vi "Driver.vi"(9 "Device Inputs FIFO":refnum<k33>, 10 "Device Outputs FIFO":refnum<k33>, 11 "Device Reference":T1 format="%.0x") -> ()   [LabVIEW 2023, in "NI 272x Resistive Simulation Custom Device Engine.lvlib"]
uses:
  NI 272x Resistive Simulation Custom Device Engine.lvlib
  <vilib>/NI VeriStand/Custom Device Tools/Custom Device Utility Library/Custom Device Utility Library.lvlib
  <vilib>/Platform/TimedLoop/XDataNode/XDataNode.xnode
  <vilib>/Platform/TimedLoop/XDataNode/nitl_modes.ctl
  <vilib>/Platform/TimedLoop/XDataNode/XDNodeRunTimeDep.lvlib
  <vilib>/Platform/TimedLoop/XDataNode/wakeup.ctl
  <vilib>/Platform/TimedLoop/XDataNode/timing_clust.ctl
  Controls/Connection control.ctl
  <vilib>/NI VeriStand/Custom Device API/Custom Device Item Ref.ctl
  <vilib>/NI VeriStand/Custom Device API/Custom Device API.lvlib
panel:
  in  "Initialization Status Notifier":refnum<notifier>
  in  "Status Notifier":refnum<notifier>
  # "Custom Device Template\nv1.0"
  # "Use this template as a starting point for creating a custom device code module. The input controls shown here are specially named controls that the system will use to provide the device loop with data. The controls are not required for the device loop to run. For instance, if the device doesn't produce any output data, then you don't need the Device Outputs FIFO control. If you do use these controls, however, they need to have these exact names to be functional."
  # "The optional status notifier element is used to notify the RT engine of the last state of the custom device, and to indicate the device has completed execution. If this control is not used, a default No Error value is returned to the system when the device finishes execution.\n\nNote: This error state is not checked until the system shuts down. Use an output status channel to send more immediate status values to the system."
  # "This optional input can be used to send the VeriStand Engine the final status of the custom device initalization process. If this control exists on the custom device front panel, the VeriStand Engine will wait for a status update before starting up. If the custom device reports an error, that will abort the execution of the current configuration in the VeriStand Engine.\n\nThis control can be deleted if the custom device does not need to send the initialization status update."
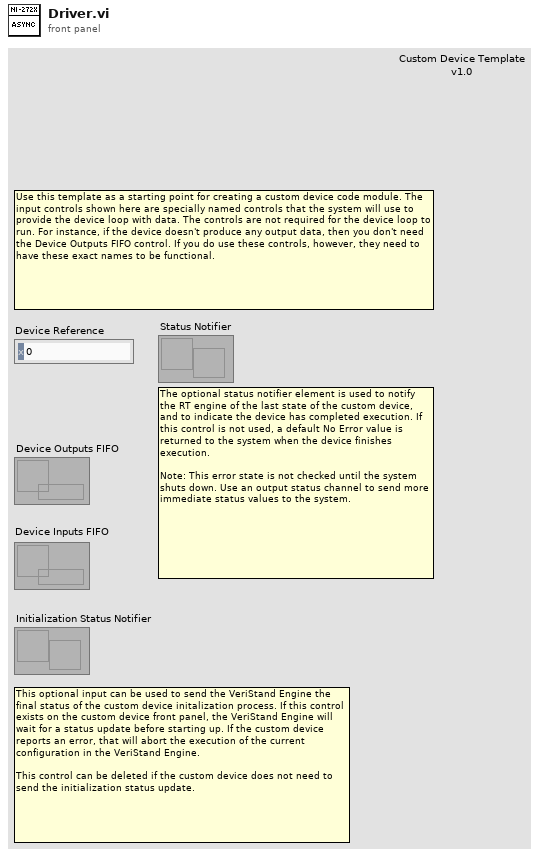
[diagram p1: front panel]
types:
  T1 = typedef "Custom Device API.lvlib/Custom Device Item Ref.ctl" = u64
  T2 = typedef "NI 272x Resistive Simulation Custom Device Engine.lvlib/Connection control.ctl" = enum16{"Connect (First Iter Only)", "Disconnect"}
  T3 = typedef "NI 272x Resistive Simulation Custom Device Engine.lvlib/Engine Run Time Data.ctl" = cluster{"Compiled Engine Data":T4, "CD In Buf":dbl[], "CD Out Buf":dbl[], "Device Outputs FIFO":refnum<k33>, "Device Inputs FIFO":refnum<k33>, "Instr":T9, "FirstIter":bool}
  T4 = typedef "NI 272x Resistive Simulation Custom Device Shared.lvlib/Compiled Engine Data.ctl" = cluster{"HW Chns":T5[], "Con Chns":T8[], "Err Idx":i32, "Late Idx":i32, "Dur Idx":i32, "DevName":string, "CD In Size":i32, "CD Out Size":i32, "TL dt":i64}
  T5 = typedef "NI 272x Resistive Simulation Custom Device Shared.lvlib/Compiled HW Channel.ctl" = cluster{"Mode":T6, "RTD":T7, "Desired Idx":i32, "Actual Idx":i32, "Last Des Val":dbl, "HW CH":string}
  T6 = typedef "NI 272x Resistive Simulation Custom Device Shared.lvlib/Channel Mode.ctl" = enum16{"Resistance", "RTD Temperature"}
  T7 = typedef "ni272x Callendar-Van Dusen RTD Parameters.ctl" = cluster{"A":dbl, "B":dbl, "C":dbl, "R0":dbl}
  T8 = typedef "NI 272x Resistive Simulation Custom Device Shared.lvlib/Compiled Connect Channel.ctl" = cluster{"Chn Idx":i32, "HW CH":string, "Is Con":bool, "HW CH+1":string}
  T9 = typedef "ni272x Reference.ctl" = refnum<k20>
  T10 = typedef "XDNodeRunTimeDep.lvlib/timing_clust.ctl" = cluster{"Expected End [f-1]":u64, "Actual End [f-1]":u64, "Finished Late? [f-1]":bool, "Expected End [i-1]":u64, "Actual End [i-1]":u64, "Finished Late? [i-1]":bool, "Expected Start [i]":u64, "Actual Start [i]":u64, "Expected Start [f]":u64, "Actual Start [f]":u64, "Source Name":string, "Structure Name":string, "Period":i64, "Deadline":i64, "Offset":i64, "Start":i64, "Priority":i32, "Timeout":i32, "Mode":T11, "Wakeup Reason":T12, "Error":errorcluster, "Source Type":string, "Secondary Source Type":string, "Global End Time":u64, "Global Start Time":u64, "Frame Duration":u64, "Iteration Duration":u64, "Assigned CPU":i32, "I/O Scan Engine Mode":u32}
  T11 = typedef "XDNodeRunTimeDep.lvlib/nitl_modes.ctl" = enum32{"No Change", "Process missed periods, maintain original phase", "Discard missed periods, maintain original phase", "Process missed periods, ignore original phase", "Discard missed periods, ignore original phase"}
  T12 = typedef "XDNodeRunTimeDep.lvlib/wakeup.ctl" = enum32{"Normal", "Aborted", "Asynchronous wakeup", "Timing source error", "Timed loop error", "Timeout"}
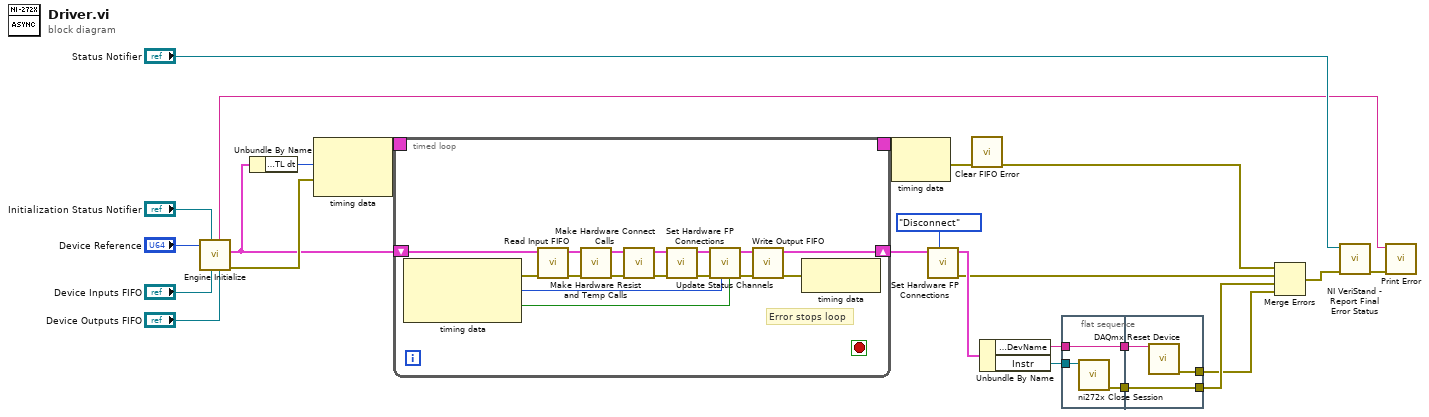
[diagram p0: block diagram]
diagram:
  n1 = call "Engine Initialize.vi"("Device Outputs FIFO"="Device Outputs FIFO", "Device Inputs FIFO"="Device Inputs FIFO", "Initialization Status Notifier"="Initialization Status Notifier", "Device Reference"="Device Reference") -> ("error out"=w19:errorcluster, "Engine Run Time Data"=w18:T3, "Device Name"=w15:string)  [unwired: 4 in, 1 out]
  n2 = Unbundle By Name(w18) -> ("Compiled Engine Data.TL dt"=w12:i64)
  n3 = node-c288(w12, w19) -> (w14:T10)
  n4 = timed-loop {
    timing: w14 -> [_]
    timing-out: [_] -> w13
    shift-right: [w39] -> w17
    shift-left: w18 -> [w40]
    stop <- _ stop-if-true
    # "Error stops loop"
    n5 = node-c288() -> (w41:errorcluster, w38:i64, w37:bool)  [unwired: 1 in]
    n6 = call "Read Input FIFO.vi"("error in (no error)"=w41, "Engine Run Time Data in"=w40) -> ("error out"=w36:errorcluster, "Engine Run Time Data out"=w32:T3)  [unwired: 8 in]
    n7 = call "Make Hardware Resist and Temp Calls.vi"("error in (no error)"=w36, "Engine Run Time Data in"=w32) -> ("error out"=w33:errorcluster, "Engine Run Time Data out"=w30:T3)  [unwired: 8 in]
    n8 = call "Make Hardware Connect Calls.vi"("error in (no error)"=w33, "Engine Run Time Data in"=w30) -> ("error out"=w31:errorcluster, "Engine Run Time Data out"=w28:T3)  [unwired: 8 in]
    n9 = call "Set Hardware FP Connections.vi"("error in (no error)"=w31, "Engine Run Time Data in"=w28) -> ("error out"=w29:errorcluster, "Engine Run Time Data out"=w27:T3)  [unwired: 8 in]
    n10 = call "Update Status Channels.vi"("Finished Late? [i-1]"=w37, "Iteration Duration"=w38, "error in (no error)"=w29, "Engine Run Time Data in"=w27) -> ("error out"=w35:errorcluster, "Engine Run Time Data out"=w34:T3)  [unwired: 6 in]
    n11 = call "Write Output FIFO.vi"("error in (no error)"=w35, "Engine Run Time Data in"=w34) -> ("error out"=w26:errorcluster, "Engine Run Time Data out"=w39:T3)  [unwired: 8 in]
    n12 = node-c288(w26) -> ()  [unwired: 1 out]
  }
  n13 = node-c288(w13) -> (w11:errorcluster)
  n14 = call "Set Hardware FP Connections.vi"("command (Connect)"=Connection_control."Disconnect", "Engine Run Time Data in"=w17) -> ("error out"=w4:errorcluster, "Engine Run Time Data out"=w9:T3)  [unwired: 8 in]
  n15 = call "Clear FIFO Error.vi"("error in (no error)"=w11) -> ("error out"=w5:errorcluster)  [unwired: 10 in]
  n16 = Unbundle By Name(w9) -> ("Compiled Engine Data.DevName"=w6:string, "Instr"=w8:T9)
  n17 = flat-sequence {
    tunnel: w8 -> [w51]
    tunnel: [w50] -> w7
    tunnel: w6 -> [w50]
    tunnel: [w49] -> w3
    tunnel: w7 -> [w54]
    tunnel: w3 -> [w53]
    tunnel: [w53] -> w2
    tunnel: [w52] -> w1
    frame #0 {
      n18 = call <instrlib>:"ni272x Close Session.vi"("instrument handle"=w51) -> ("error out"=w49:errorcluster)  [unwired: 2 in, 8 out]
    }
    frame #1 {
      n19 = call <vilib>:"DAQmx Reset Device.vi"("device in"=w54) -> ("error out"=w52:errorcluster)  [unwired: 1 in, 13 out]
    }
  }
  n20 = Merge Errors(w5, w4, w2, w1) -> (w23:errorcluster)
  n21 = call <vilib>:"NI VeriStand - Report Final Error Status.vi"("error in (no error)"=w23, "Status Notifier"="Status Notifier") -> ("error out"=w16:errorcluster)  [unwired: 1 in, 8 out]
  n22 = call "Print Error.vi"("error out"=w16, "Your code's public name"=w15) -> ()  [unwired: 9 in]
